vi "Close.vi"(8 "error in (no error)":errorcluster, 11 "Keysight 5700C in":refnum<class "Keysight 5700C.lvclass">) -> (0 "error out":errorcluster, 3 "Keysight 5700C out":refnum<class "Keysight 5700C.lvclass">)   [LabVIEW 2021, in "Concrete.lvlib" / "Keysight 5700C.lvclass"]
uses:
  Keysight 5700C.lvclass
  Keysight 5700C.lvclass/Keysight 5700C.ctl
  Harware Abstraction/AnalogIO/Power Supply.lvclass
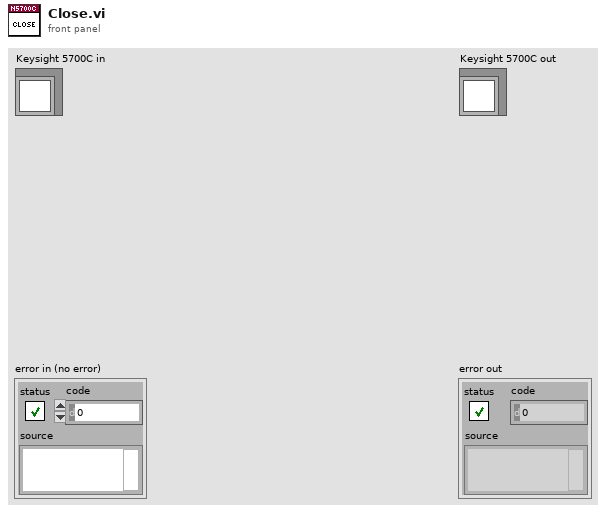
[diagram p1: front panel]
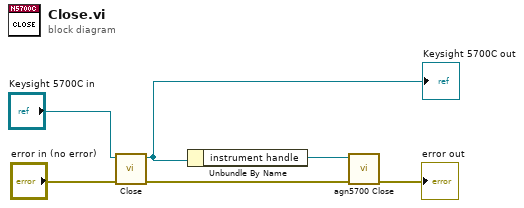
[diagram p0: block diagram]
diagram:
  n1 = call-parent "Close.vi"("error in (no error)"="error in (no error)", "Instrument in"="Keysight 5700C in") -> ("error out"=w3:errorcluster, "Instrument out"=w4:refnum<class "Keysight 5700C.lvclass">)  [unwired: 8 in]
  "Keysight 5700C out" <- w4
  n2 = Unbundle By Name(w4) -> ("instrument handle"=w2:refnum<k15>)
  n3 = call <instrlib>:"agn5700 Close.vi"("error in (no error)"=w3, "instrument handle"=w2) -> ("error out"=→"error out":errorcluster)  [unwired: 9 out]
